vi "Run Filter.vi"(8 "error in (no error)":errorcluster, 10 "resource entries in":T1[](array[typedef]) {"FPGA CD Ref" format="%.0x"; "reserver" format="%.0x"}, 11 "Filter in":refnum<class "Filter.lvclass">) -> (0 "error out":errorcluster, 2 "resource entries out":T1[](array[typedef]) {"FPGA CD Ref" format="%.0x"; "reserver" format="%.0x"})   [LabVIEW 2016, in "Filter.lvclass"]
uses:
  Filter.lvclass
  Server/viz_entry.ctl
  <vilib>/NI Veristand/Custom Device API/Custom Device Item Ref.ctl
  Boolean Filter Parent/Boolean Filter.lvclass
  <vilib>/NI VeriStand/Custom Device API/Custom Device API.lvlib
  Server/RM.Server.lvlib
panel:
  in  "Boolean Filter.lvclass":refnum<class "Boolean Filter.lvclass">
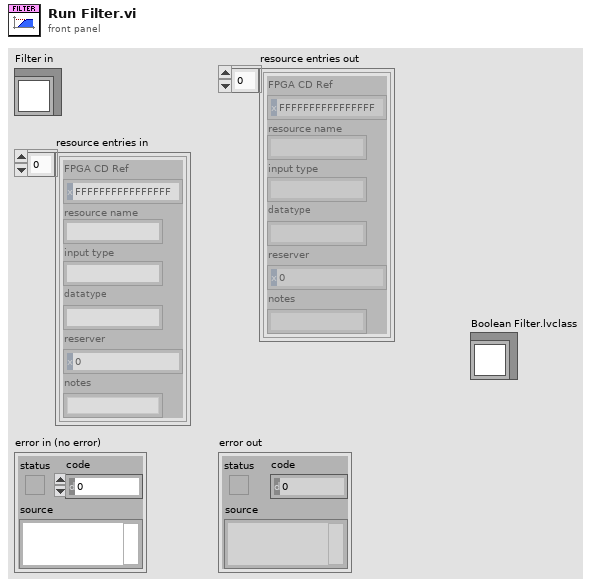
[diagram p1: front panel]
types:
  T1 = typedef "RM.Server.lvlib/viz_entry.ctl" = cluster{"FPGA CD Ref":T2, "resource name":string, "input type":string, "datatype":string, "reserver":T2, "notes":string}
  T2 = typedef "Custom Device API.lvlib/Custom Device Item Ref.ctl" = u64
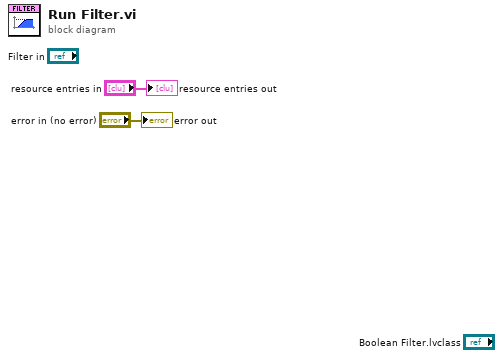
[diagram p0: block diagram]
diagram:
  "error out" <- "error in (no error)"
  "resource entries out" <- "resource entries in"
